vi "main.vi"() -> ()   [LabVIEW 2010]
uses:
  object_parameters.ctl
  common/classes/ImageCollection/ImageCollection/ImageCollection.lvclass
  common/classes/Image/Image/Image.lvclass
panel:
  in  "Path":path=path "C:/helioscan/tools/PSFAnalyzerMH110526/test stack/150x512x512.tif"
  in  "stop":bool
  in  "analyze z":bool
  in  "select % threshold":dbl=0.1
  in  "settings for z":T1={"Objects"=0, "Threshold"=6700, "Reject Border"=TRUE, "Fill Holes"=FALSE, "Min Object Size"=TRUE, "Min Size"=30, "Max Object Size"=FALSE, "Max Size"=100, "Show Search Area"=FALSE, "Show Center"=FALSE, "Show Bounding Box"=TRUE} {"Objects" items=["Bright Objects", "Dark Objects"]}
  in  "settings for xy":T1={"Objects"=0, "Threshold"=6700, "Reject Border"=TRUE, "Fill Holes"=FALSE, "Min Object Size"=TRUE, "Min Size"=30, "Max Object Size"=FALSE, "Max Size"=100, "Show Search Area"=FALSE, "Show Center"=FALSE, "Show Bounding Box"=TRUE} {"Objects" items=["Bright Objects", "Dark Objects"]}
  in  "expected size in pixels z":dbl=3.0
  out "regions found with fit parameters 2":T2[][](array[typedef])
  out "regions found with fit parameters":T2[][](array[typedef])
  in  "load images":bool
  in  "expected size in pixels xy":dbl=3.0
  in  "analyze xy":bool
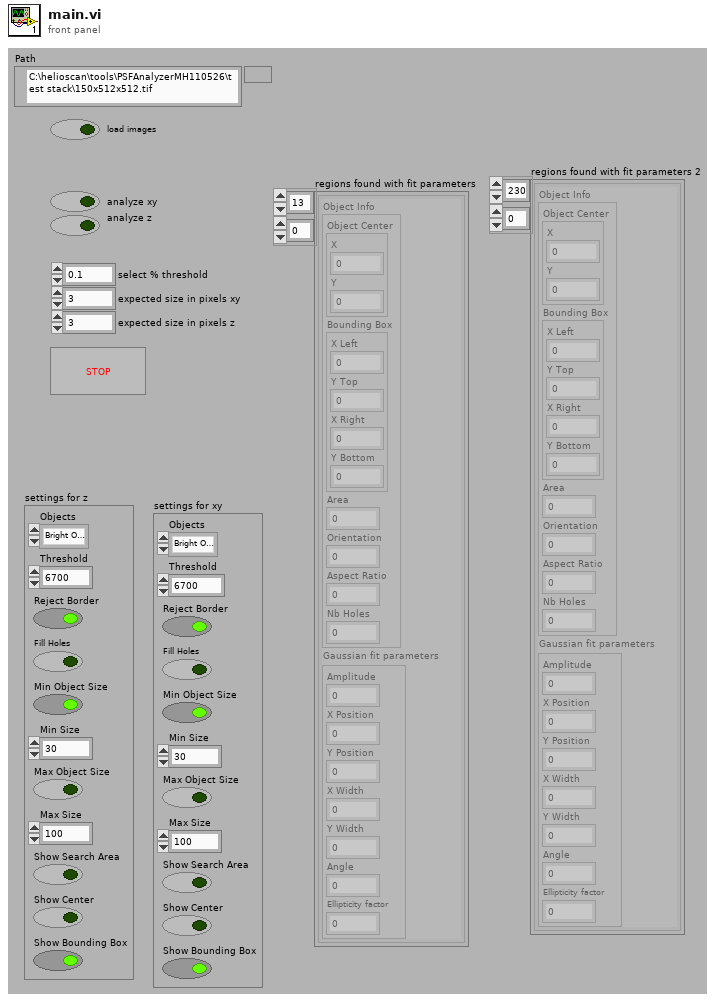
[diagram p1: front panel]
types:
  T1 = cluster{"Objects":u16, "Threshold":i32, "Reject Border":bool, "Fill Holes":bool, "Min Object Size":bool, "Min Size":i32, "Max Object Size":bool, "Max Size":i32, "Show Search Area":bool, "Show Center":bool, "Show Bounding Box":bool}
  T2 = typedef "object_parameters.ctl" = cluster{"Object Info":cluster{"Object Center":cluster{"X":sgl, "Y":sgl}, "Bounding Box":cluster{"X Left":i32, "Y Top":i32, "X Right":i32, "Y Bottom":i32}, "Area":sgl, "Orientation":sgl, "Aspect Ratio":sgl, "Nb Holes":i32}, "Gaussian fit parameters":cluster{"Amplitude":dbl, "X Position":dbl, "Y Position":dbl, "X Width":dbl, "Y Width":dbl, "Angle":dbl, "Ellipticity factor":dbl}}
  T3 = typedef "Image Type" = u32
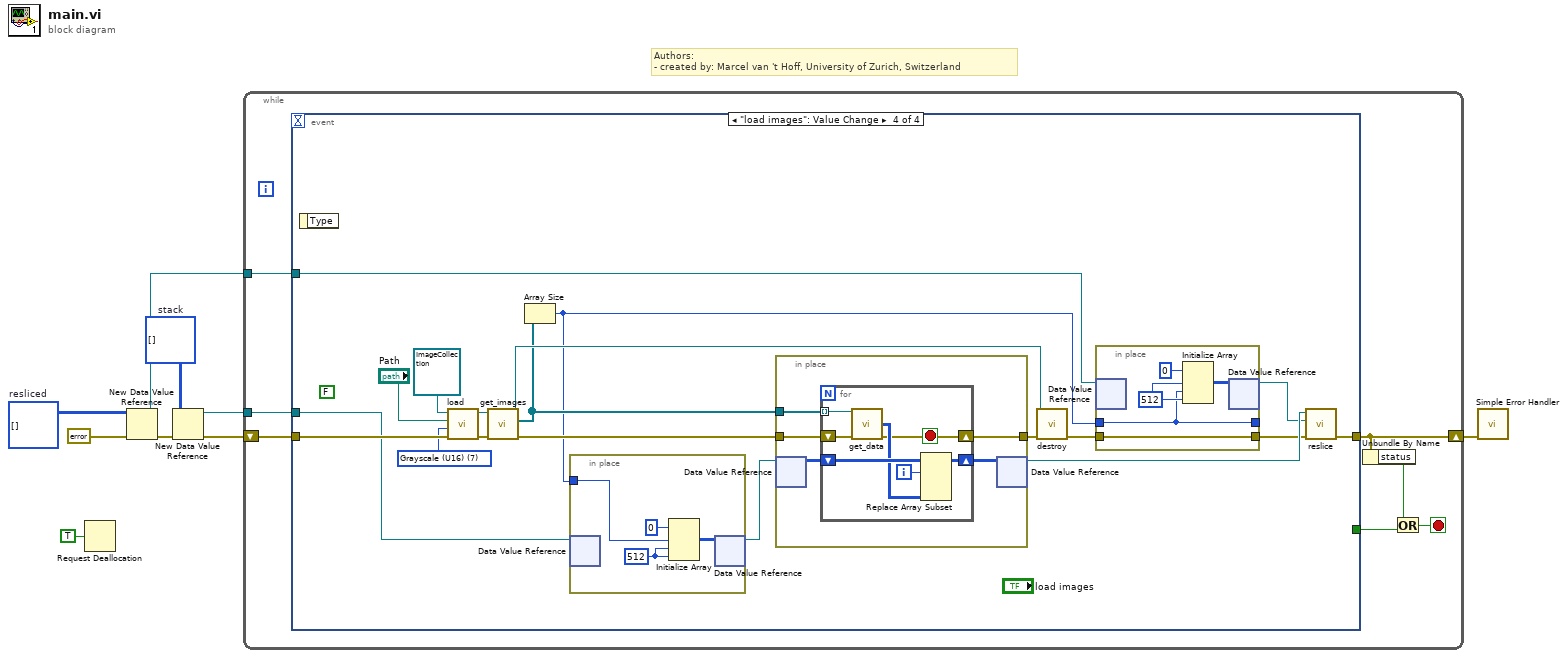
[diagram p0: block diagram]
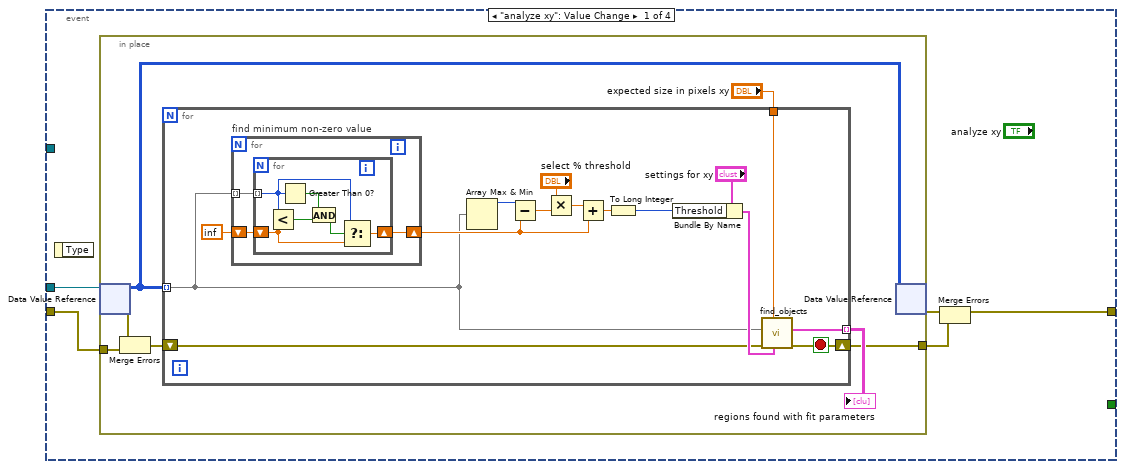
[diagram p2: hidden frame]
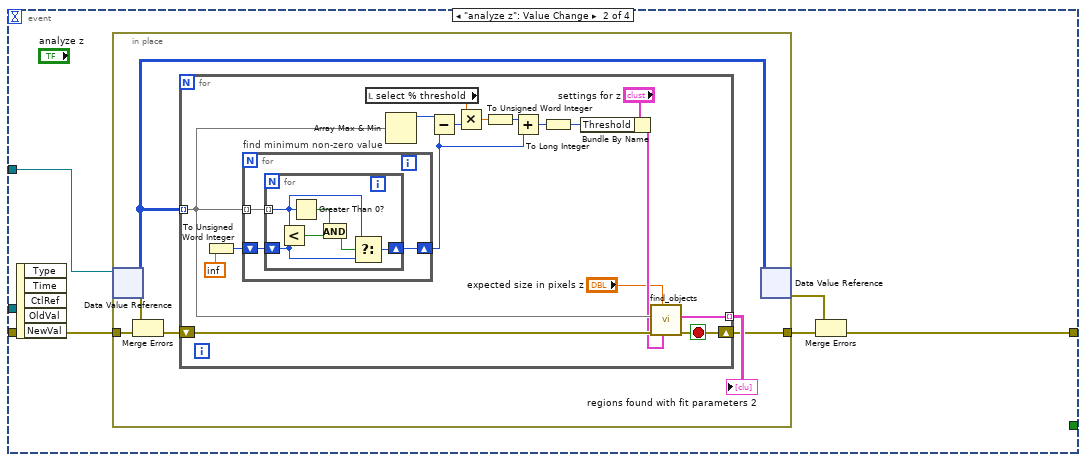
[diagram p3: hidden frame]
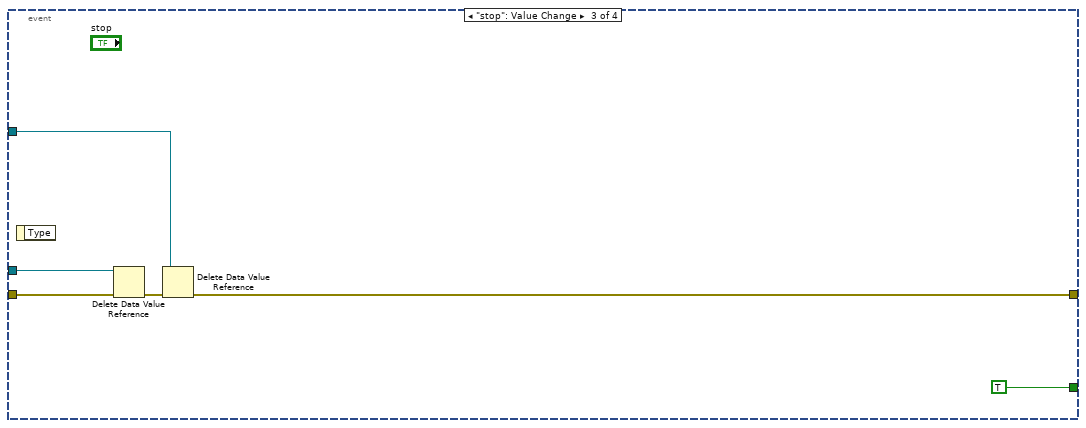
[diagram p4: hidden frame]
diagram:
  w5 = u16[][][] []  # stack
  w8 = u16[][][] []  # resliced
  # "Authors: \n- created by: Marcel van 't Hoff, University of Zurich, Switzerland"
  n1 = Request Deallocation(TRUE ("flag")) -> ()
  n2 = New Data Value Reference(data value=w8, error in=errorcluster {"status"=FALSE, "code"=0, "source"=""} ("error out")) -> (data value reference=w7:refnum<data-value>, error out=w4:errorcluster)
  n3 = New Data Value Reference(data value=w5, error in=w4) -> (data value reference=w2:refnum<data-value>, error out=w3:errorcluster)
  n4 = while {
    shift-right: [w15] -> w1
    shift-left: w3 -> [w16]
    tunnel: w7 -> [w12]
    tunnel: w2 -> [w11]
    stop <- w13 stop-if-true
    n5 = event shown="[3] \"load images\": Value Change" {
      selector: _ -> [_ _ _ _]
      dyn-events: _ -> [_ _ _ _]
      timeout: _ -> [_ _ _ _]
      tunnel: [w17 w53 w91 w114] -> w15
      tunnel: w16 -> [w21 w57 w92 w113]
      tunnel: w12 -> [_ w56 w95 w102]
      tunnel: w11 -> [w20 _ w94 w112]
      tunnel: [_ _ TRUE _] -> w10
      event "analyze xy": Value Change {
        n6 = event-data() -> ()  [unwired: 1 in, 1 out]
        n7 = in-place {
          in-place-border: w21 -> [w24]
          in-place-border: [w26] -> w19
          n8 = in-place-dvr #1(w20) -> (w22:u16[][][], w25:errorcluster)
          n9 = Merge Errors(w25, w24) -> (w23:errorcluster)
          n10 = for {
            tunnel: w22 -> [w30] mode=indexing
            tunnel: "expected size in pixels xy" -> [w36]
            tunnel: [w32] -> w27 mode=indexing
            shift-right: [w29] -> w26
            shift-left: w23 -> [w31]
            stop <- w29 stop-if-true
            n11 = for "find minimum non-zero value" {
              tunnel: w30 -> [w46] mode=indexing
              shift-right: [w44] -> w37
              shift-left: inf -> [w45]
              n12 = for {
                tunnel: w46 -> [w50] mode=indexing
                shift-right: [w52] -> w44
                shift-left: w45 -> [w51]
                n13 = Less?(x=w50, y=w51) -> (x < y?=w48:bool)
                n14 = Greater Than 0?(x=w50) -> (x > 0?=w49:bool)
                n15 = And(x=w49, y=w48) -> (x .and. y?=w47:bool)
                n16 = Select(t=w50, s=w47, f=w51) -> (s? t:f=w52:dbl)
              }
            }
            n17 = Array Max & Min(array=w30) -> (max value=w39:u16)  [unwired: 3 out]
            n18 = Subtract(x=w39, y=w37) -> (x-y=w40:dbl)
            n19 = Multiply ("select 5%")(x="select % threshold", y=w40) -> (x*y=w42:dbl)
            n20 = Add(x=w42, y=w37) -> (x+y=w43:dbl)
            n21 = To Long Integer(number=w43) -> (32bit integer=w34:i32)
            n22 = Bundle By Name(cluster="settings for xy", "Threshold"=w34) -> (w33:T1)
            n23 = call "find_objects.vi"("objects finding parameters in"=w33, "expected size in pixels"=w36, "error in"=w31, "array in"=w30) -> ("error out"=w29:errorcluster, "regions found with fit parameters"=w32:T2[])  [unwired: 6 in]
          }
          "regions found with fit parameters" <- w27
          n24 = in-place-dvr #1(w22) -> (w18:errorcluster)  [unwired: 1 out]
        }
        n25 = Merge Errors(w18, w19) -> (w17:errorcluster)
      }
      event "analyze z": Value Change {
        n26 = event-data() -> ()  [unwired: 1 in, 5 out]
        n27 = in-place {
          in-place-border: w57 -> [w61]
          in-place-border: [w58] -> w54
          n28 = in-place-dvr #2(w56) -> (w59:u16[][][], w62:errorcluster)
          n29 = Merge Errors(w62, w61) -> (w60:errorcluster)
          n30 = for {
            tunnel: w59 -> [w71] mode=indexing
            shift-right: [w79] -> w58
            shift-left: w60 -> [w80]
            tunnel: [w78] -> w63 mode=indexing
            stop <- w79 stop-if-true
            n31 = To Unsigned Word Integer(number=inf) -> (unsigned 16bit integer=w66:u16)
            n32 = for "find minimum non-zero value" {
              tunnel: w71 -> [w83] mode=indexing
              shift-right: [w81] -> w72
              shift-left: w66 -> [w82]
              n33 = for {
                tunnel: w83 -> [w87] mode=indexing
                shift-right: [w89] -> w81
                shift-left: w82 -> [w88]
                n34 = Less?(x=w87, y=w88) -> (x < y?=w85:bool)
                n35 = Greater Than 0?(x=w87) -> (x > 0?=w86:bool)
                n36 = And(x=w86, y=w85) -> (x .and. y?=w84:bool)
                n37 = Select(t=w87, s=w84, f=w88) -> (s? t:f=w89:u16)
              }
            }
            n38 = local read "select % threshold"() -> (w70:dbl)
            n39 = Array Max & Min(array=w71) -> (max value=w73:u16)  [unwired: 3 out]
            n40 = Subtract(x=w73, y=w72) -> (x-y=w76:u16)
            n41 = Multiply ("select 5%")(x=w70, y=w76) -> (x*y=w75:dbl)
            n42 = To Unsigned Word Integer(number=w75) -> (unsigned 16bit integer=w65:u16)
            n43 = Add(x=w65, y=w72) -> (x+y=w74:u16)
            n44 = To Long Integer(number=w74) -> (32bit integer=w69:i32)
            n45 = Bundle By Name(cluster="settings for z", "Threshold"=w69) -> (w67:T1)
            n46 = call "find_objects.vi"("objects finding parameters in"=w67, "expected size in pixels"="expected size in pixels z", "error in"=w80, "array in"=w71) -> ("error out"=w79:errorcluster, "regions found with fit parameters"=w78:T2[])  [unwired: 6 in]
          }
          "regions found with fit parameters 2" <- w63
          n47 = in-place-dvr #2(w59) -> (w55:errorcluster)  [unwired: 1 out]
        }
        n48 = Merge Errors(w55, w54) -> (w53:errorcluster)
      }
      event "stop": Value Change {
        n49 = event-data() -> ()  [unwired: 1 in, 1 out]
        n50 = Delete Data Value Reference(data value reference=w94, error in=w92) -> (error out=w93:errorcluster)  [unwired: 1 out]
        n51 = Delete Data Value Reference(data value reference=w95, error in=w93) -> (error out=w91:errorcluster)  [unwired: 1 out]
      }
      event "load images": Value Change {
        w108 = T3 7 items=["Grayscale (U8)", "Grayscale (I16)", "Grayscale (SGL)", "Complex (CSG)", "RGB (U32)", "HSL (U32)", "RGB (U64)", "Grayscale (U16)"] ("Image Type")
        (unwired) FALSE
        n52 = event-data() -> ()  [unwired: 1 in, 1 out]
        n53 = call "load.vi"("error in (no error)"=w113, "Image Type"=w108, "path in"="Path", "ImageCollection in"=refnum<class "ImageCollection.lvclass"> refnum) -> ("error out"=w110:errorcluster, "ImageCollection out"=w111:refnum<class "ImageCollection.lvclass">)  [unwired: 3 in, 3 out]
        n54 = call-dynamic "get_images.vi"("error in (no error)"=w110, "ImageCollection.lvclass in"=w111) -> ("error out"=w100:errorcluster, "images"=w105:refnum<class "Image.lvclass">[], "ImageCollection.lvclass out"=w107:refnum<class "ImageCollection.lvclass">)  [unwired: 7 in]
        n55 = Array Size(array=w105) -> (size(s)=w99:i32)
        n56 = in-place {
          in-place-border: w99 -> [w134]
          w133 = 512
          n57 = in-place-dvr #3(w112) -> ()  [unwired: 2 out]
          n58 = Initialize Array(u16 0, w134, w133, w133) -> (w132:u16[][][])
          n59 = in-place-dvr #3(w132) -> (w106:refnum<data-value>)  [unwired: 1 out]
        }
        n60 = in-place {
          in-place-border: w105 -> [w124]
          in-place-border: [w121] -> w104
          in-place-border: w100 -> [w120]
          n61 = in-place-dvr #4(w106) -> (w123:u16[][][])  [unwired: 1 out]
          n62 = for {
            tunnel: w124 -> [w131] mode=indexing
            shift-right: [w128] -> w122
            shift-left: w123 -> [w129]
            shift-right: [w125] -> w121
            shift-left: w120 -> [w127]
            i -> [w130]
            stop <- w125 stop-if-true
            n63 = call-dynamic "get_data.vi"("Image in"=w131, "error in (no error)"=w127) -> ("Image Pixels (U16)"=w126:u16[][], "error out"=w125:errorcluster)  [unwired: 5 in, 7 out]
            n64 = Replace Array Subset(array=w129, new element=w126, index (dim 0)=w130) -> (w128:u16[][][])  [unwired: 2 in]
          }
          n65 = in-place-dvr #4(w122) -> (w103:refnum<data-value>)  [unwired: 1 out]
        }
        n66 = call-dynamic "destroy.vi"("error in (no error)"=w104, "ImageCollection in"=w107) -> ("error out"=w98:errorcluster)  [unwired: 8 in, 1 out]
        n67 = in-place {
          in-place-border: w99 -> [w116]
          in-place-border: [w116] -> _
          in-place-border: [w115] -> w97
          in-place-border: w98 -> [w115]
          w117 = 512
          n68 = in-place-dvr #5(w102) -> ()  [unwired: 2 out]
          n69 = Initialize Array(u16 0, w117, w116, w117) -> (w118:u16[][][])
          n70 = in-place-dvr #5(w118) -> (w101:refnum<data-value>)  [unwired: 1 out]
        }
        n71 = call "reslice.vi"("error in"=w97, "data value reference reslice"=w101, "data value reference stack"=w103) -> ("error out"=w114:errorcluster)  [unwired: 6 in, 2 out]
      }
    }
    n72 = Unbundle By Name(w15) -> ("status"=w14:bool)
    n73 = Or(x=w14, y=w10) -> (x .or. y?=w13:bool)
  }
  n74 = call <vilib>:"Simple Error Handler.vi"("error in (no error)"=w1) -> ()  [unwired: 4 in, 5 out]
